vi "MessageName.vi"() -> (2 "MessageName":string)   [LabVIEW 2020, in "GroupData.lvlib"]
uses:
  GroupData.lvlib
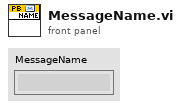
[diagram p1: front panel]
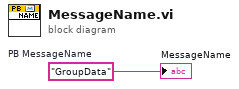
[diagram p0: block diagram]
diagram:
  w1 = "GroupData"  # PB MessageName
  "MessageName" <- w1
